vi "Configure Math (Unary Operation).vi"(0 "VISA resource name":refnum<visa-resource-name>, 1 "Enable Math Channel (T:Enable)":bool=TRUE, 2 "Number of Averages (16)":i32=16, 3 "Enable Low Pass and Phase Align Filter (T: Enable)":bool=TRUE, 5 "Math Channel (0: Function 1)":i32(ring) items=["Function 1", "Function 2", "Function 3", "Function 4", "Function 5", "Function 6", "Function 7", "Function 8", "Function 9", "Function 10", "Function 11", "Function 12", "Function 13", "Function 14", "Function 15", "Function 16"], 7 "Math Operand (1: Channel 1)":i32(ring)=1 items=["Channel 1"=1, "Channel 2"=2, "Channel 3"=3, "Channel 4"=4, "Function 1"=5, "Function 2"=6, "Function 3"=7, "Function 4"=8, "Memory 1"=9, "Memory 2"=10, "Memory 3"=11, "Memory 4"=12, "Differential 1"=61, "Differential 2"=62, "Common 1"=71, "Common 2"=72], 9 "Math Operation (0: Average)":i32(ring) items=["Average", "Differentiate", "FFT Magnitude", "FFT Phase", "High Pass Filter", "Integrate", "Invert", "Low Pass Filter", "Magnify", "Max", "Min", "Smooth", "Square Root", "Square"], 11 "error in (no error)":errorcluster, 12 "Bandwidth (3.5E+8)":dbl=350000000.0, 13 "Smoothing Points (5)":i32=5) -> (4 "VISA resource name out":refnum<visa-resource-name>, 15 "error out":errorcluster)   [LabVIEW 2013, in "Agilent 90000 Series.lvlib"]
doc: "Creates a mathematical expression with one operand."
uses:
  Agilent 90000 Series.lvlib
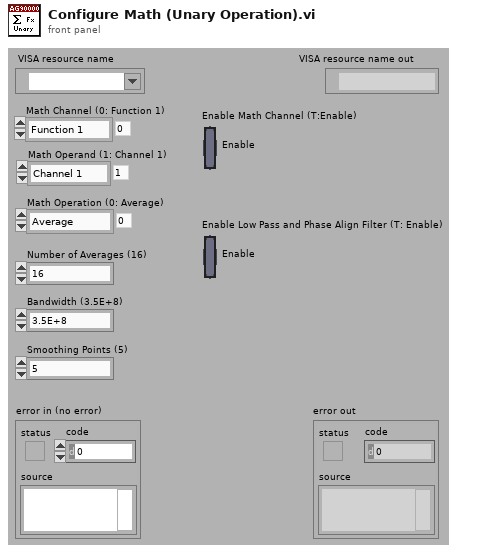
[diagram p1: front panel]
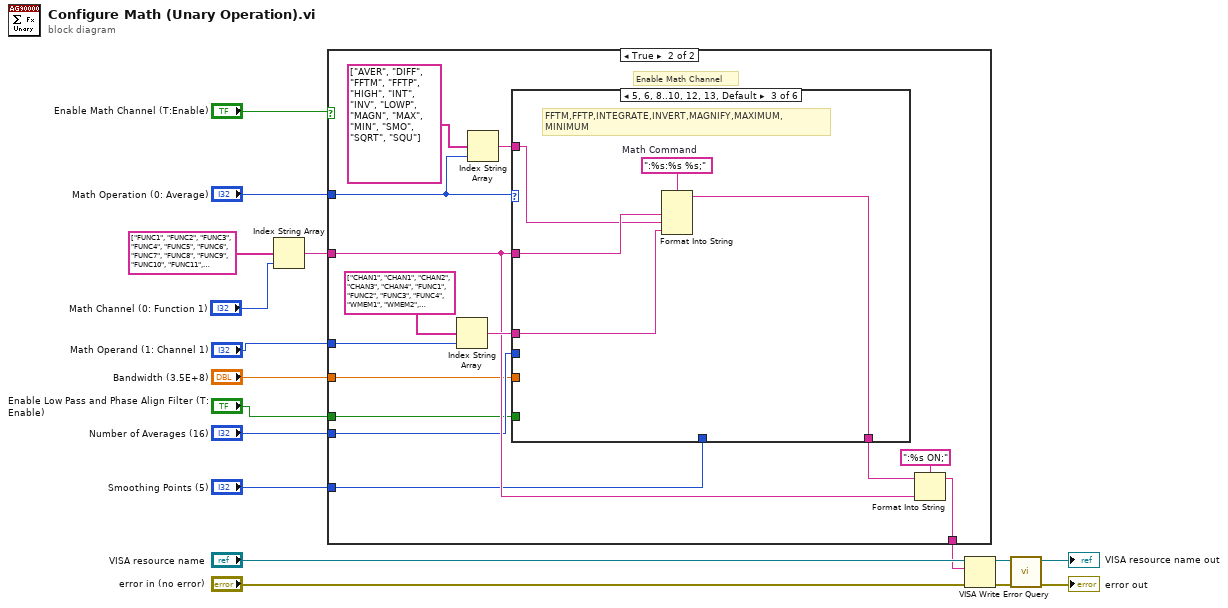
[diagram p0: block diagram]
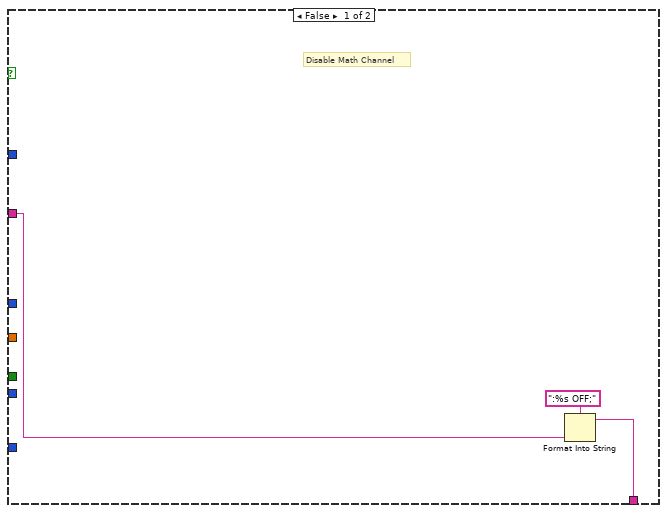
[diagram p2: hidden frame]
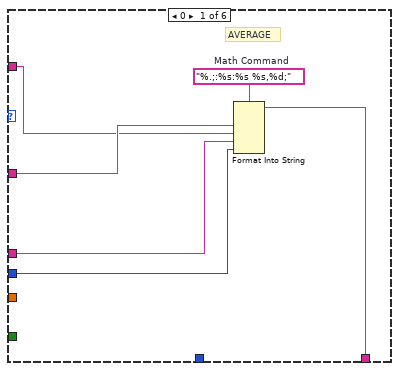
[diagram p3: hidden frame]
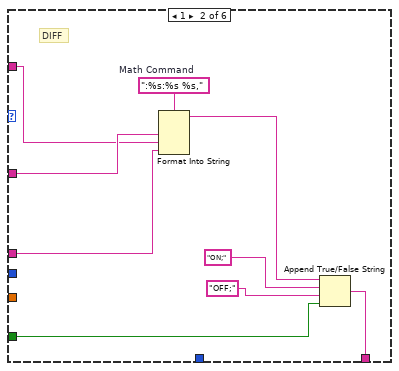
[diagram p4: hidden frame]
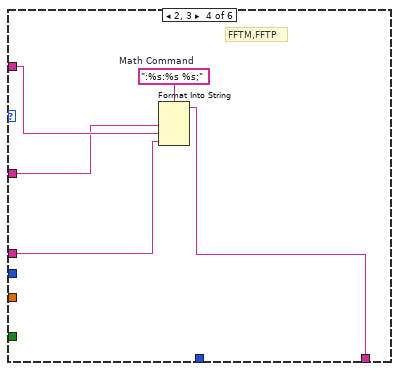
[diagram p5: hidden frame]
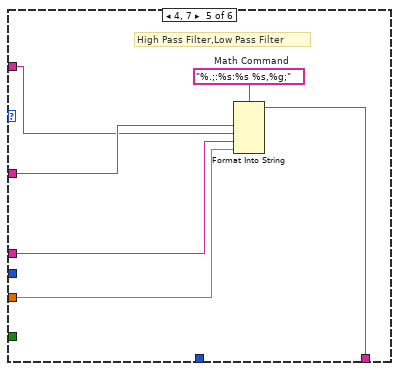
[diagram p6: hidden frame]
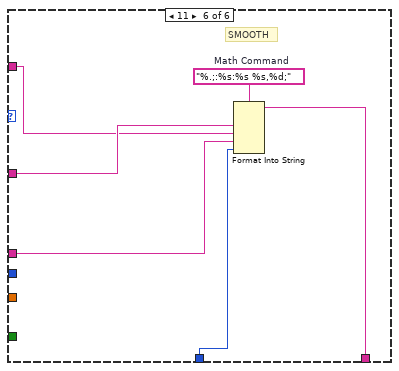
[diagram p7: hidden frame]
diagram:
  n1 = Index String Array(1:"Math Channel (0: Function 1)", 2:string[] ["FUNC1", "FUNC2", "FUNC3", "FUNC4", "FUNC5", "FUNC6", "FUNC7", "FUNC8", "FUNC9", "FUNC10", "FUNC11", "FUNC12", "FUNC13", "FUNC14", "FUNC15", "FUNC16"] ("string array")) -> (0:w11:string)  [unwired: 1 out]
  n2 = case shown="True" "Enable Math Channel (T:Enable)" {
    tunnel: w11 -> [w19 w29]
    tunnel: [w18 w28] -> w9
    tunnel: "Number of Averages (16)" -> [_ w27]
    tunnel: "Enable Low Pass and Phase Align Filter (T: Enable)" -> [_ w26]
    tunnel: "Math Operand (1: Channel 1)" -> [_ w25]
    tunnel: "Math Operation (0: Average)" -> [_ w24]
    tunnel: "Bandwidth (3.5E+8)" -> [_ w23]
    tunnel: "Smoothing Points (5)" -> [_ w22]
    frame False {
      # "Disable Math Channel"
      n3 = Format Into String(format string=":%s OFF;", w19) -> (resulting string=w18:string)  [unwired: 2 in, 1 out]
    }
    frame True {
      # "Enable Math Channel"
      n4 = Index String Array(1:w25, 2:string[] ["CHAN1", "CHAN1", "CHAN2", "CHAN3", "CHAN4", "FUNC1", "FUNC2", "FUNC3", "FUNC4", "WMEM1", "WMEM2", "WMEM3", "WMEM4", "AUX", "LINE", "CLOC", "MTR", "MSP", "EQU", "NONE", "DIG0", "DIG1", "DIG2", "DIG3", "DIG4", "DIG5", "DIG6", "DIG7", "DIG8", "DIG9", "DIG10", "DIG11", "DIG12", "DIG13", "DIG14", "DIG15", "", "", "", "", "", "POD1", "POD2", "", "", "", "", "", "", "", "", "BUS1", "BUS2", "BUS3", "BUS4", "", "", "", "", "", "", "DIFF1", "DIFF2", "", "", "", "", "", "", "", "", "COMM3", "COMM4"]) -> (0:w32:string)  [unwired: 1 in]
      n5 = Index String Array(1:w24, 2:string[] ["AVER", "DIFF", "FFTM", "FFTP", "HIGH", "INT", "INV", "LOWP", "MAGN", "MAX", "MIN", "SMO", "SQRT", "SQU"]) -> (0:w33:string)  [unwired: 1 out]
      n6 = case shown="5, 6, 8..10, 12, 13, Default" w24 {
        tunnel: w29 -> [w40 w49 w54 w56 w65 w71]
        tunnel: w33 -> [w39 w48 w53 w59 w64 w70]
        tunnel: w32 -> [w38 w47 w52 w58 w63 w69]
        tunnel: [w36 w44 w50 w55 w61 w67] -> w31
        tunnel: w27 -> [w35 _ _ _ _ _]
        tunnel: w26 -> [_ w41 _ _ _ _]
        tunnel: w23 -> [_ _ _ _ w60 _]
        tunnel: w22 -> [_ _ _ _ _ w66]
        frame 0 {
          w37 = "%.;:%s:%s %s,%d;"  # Math Command
          # "AVERAGE"
          n7 = Format Into String(format string=w37, w40, w39, w38, w35) -> (resulting string=w36:string)  [unwired: 2 in, 1 out]
        }
        frame 1 {
          w46 = ":%s:%s %s,"  # Math Command
          # "DIFF"
          n8 = Format Into String(format string=w46, w49, w48, w47) -> (resulting string=w45:string)  [unwired: 2 in, 1 out]
          n9 = Append True/False String(1:w41, 2:"OFF;" ("true string"), 3:"ON;" ("true string"), 4:w45) -> (0:w44:string)
        }
        frame 5, 6, 8..10, 12, 13, Default {
          w51 = ":%s:%s %s;"  # Math Command
          # "FFTM,FFTP,INTEGRATE,INVERT,MAGNIFY,MAXIMUM,\nMINIMUM"
          n10 = Format Into String(format string=w51, w54, w53, w52) -> (resulting string=w50:string)  [unwired: 2 in, 1 out]
        }
        frame 2, 3 {
          w57 = ":%s:%s %s;"  # Math Command
          # "FFTM,FFTP"
          n11 = Format Into String(format string=w57, w56, w59, w58) -> (resulting string=w55:string)  [unwired: 2 in, 1 out]
        }
        frame 4, 7 {
          w62 = "%.;:%s:%s %s,%g;"  # Math Command
          # "High Pass Filter,Low Pass Filter"
          n12 = Format Into String(format string=w62, w65, w64, w63, w60) -> (resulting string=w61:string)  [unwired: 2 in, 1 out]
        }
        frame 11 {
          w68 = "%.;:%s:%s %s,%d;"  # Math Command
          # "SMOOTH"
          n13 = Format Into String(format string=w68, w71, w70, w69, w66) -> (resulting string=w67:string)  [unwired: 2 in, 1 out]
        }
      }
      n14 = Format Into String(format string=":%s ON;", initial string=w31, w29) -> (resulting string=w28:string)  [unwired: 1 in, 1 out]
    }
  }
  n15 = VISA Write(VISA resource name="VISA resource name", write buffer=w9, error in (no error)="error in (no error)") -> (VISA resource name out=w13:refnum<visa-resource-name>, error out=w12:errorcluster)  [unwired: 1 out]
  n16 = call "Error Query.vi"("error in (no error)"=w12, "VISA resource name"=w13) -> ("error out"=→"error out":errorcluster, "VISA resource name out"=→"VISA resource name out":refnum<visa-resource-name>)  [unwired: 8 out]
